vi "Ion Sniffer NXG.vi"() -> ()   [LabVIEW 2018]
uses:
  Type Defs/Main States.ctl
  Type Defs/Open IPF.ctl
  Type Defs/Log Command.ctl
  Type Defs/RT Command.ctl
  FGVs/Global Variables.vi
  <vilib>/Utility/config.llb/Read Key (Path).vi
  <vilib>/Utility/config.llb/Write Key (Path).vi
  <vilib>/Utility/config.llb/Read Key (String).vi
  <vilib>/Utility/config.llb/Write Key (String).vi
  <vilib>/Utility/config.llb/Read Key (Boolean).vi
  <vilib>/Utility/error.llb/Error Cluster From Error Code.vi
  <vilib>/ErrorRing/Error Ring.xnode
  <vilib>/Utility/config.llb/NI_LVConfig.lvlib
panel:
  out "ItemTag":string
  in  "Stop":bool
  out "Error Out":errorcluster
  in  "Display":bool
  in  "Acquisition":bool
  in  "Tuning":bool
  in  "Diagnostics":bool
  in  "Configuration":bool
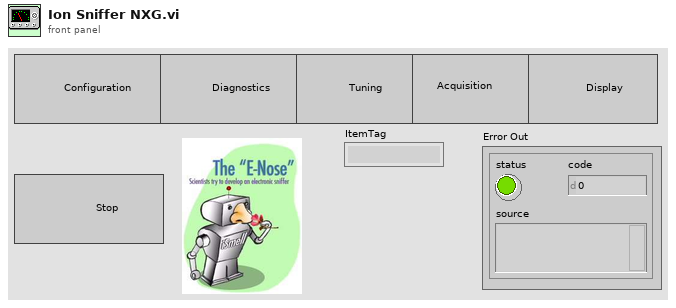
[diagram p1: front panel]
types:
  T1 = typedef "Main States.ctl" = enum16{"Initialize", "Init 2", "RT Stauts", "Exit"}
  T2 = typedef "Log Command.ctl" = enum16{"Close", "Write", "Open", "No Command"}
  T3 = typedef "Open IPF.ctl" = enum16{"Init", "Create IPF"}
  T4 = typedef "RT Command.ctl" = enum16{"xml Start Run", "xml Start Actual Run", "xml Stop Run", "xml Runtime Update", "xml Get Status", "xml Get Table", "xml Set Table", "xml Get Configuration", "xml System Status", "xml Set LC Input Logic", "xml Get Data", "xml Get Info", "Start", "StartActualRun", "Stop", "Runtime Update", "Get Data", "Get Info", "Get Status", "Get Param", "Get Config", "Get Table", "Read ADC", "Set Oscillator", "Update Config", "Update Table", "Set All Pol", "Set Pol and DC", "Set Max Mass", "Toggle RP", "Toggle EL", "Set PIC", "Initialize Turbo", "Send Turbo Comm", "Close Turbo", "P1", "P2", "P3", "Send Serial", "Set LC Out", "Get LC In", "Read VAC", "Test Table", "Toggle Power", "Get Startup", "Set Startup", "Get ADC Table", "Set ADC Table", "Get Brief Status", "Get Detail Status", "Auxiliary Update", "Set CC Logics", "Set CC Input Logics", "Ignore Error", "invalid"}
  T5 = typedef "NI_LVConfig.lvlib/Config Data RefNum.ctl" = refnum<k1>
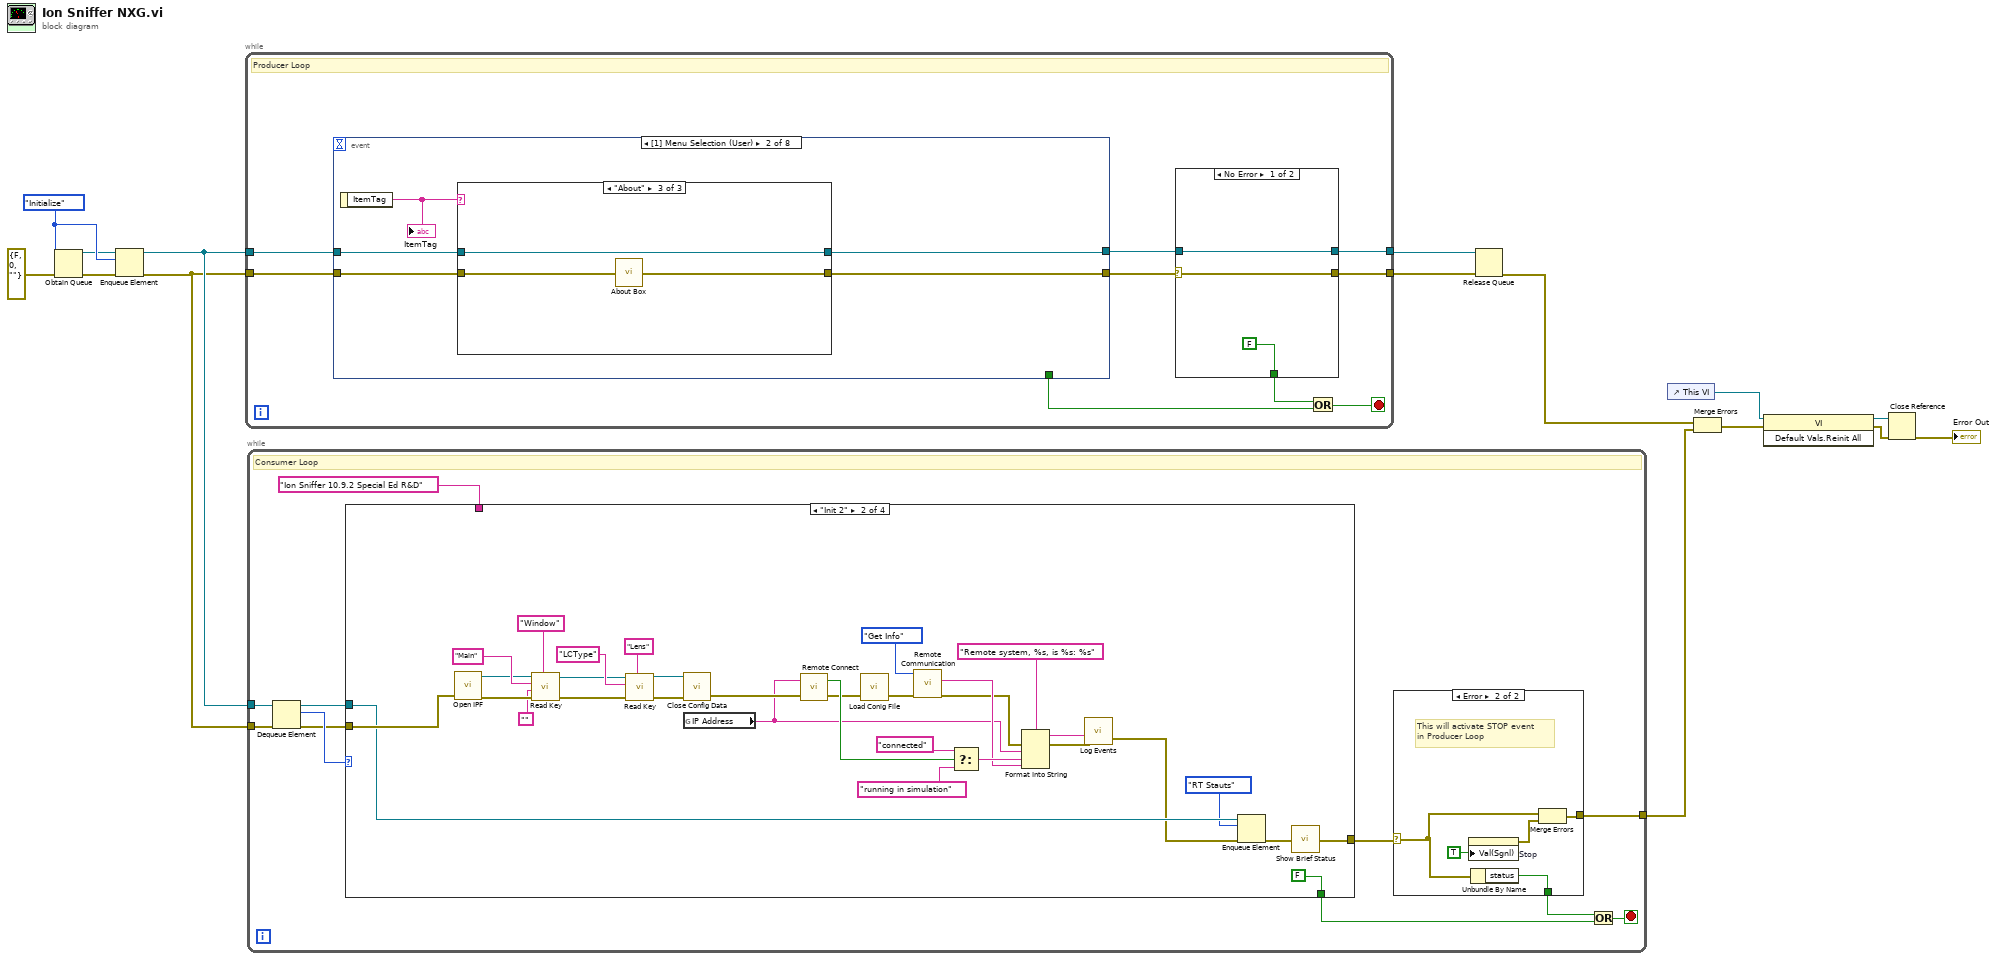
[diagram p0: block diagram]
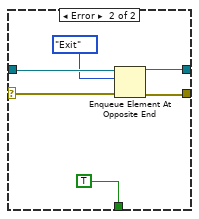
[diagram p2: hidden frame]
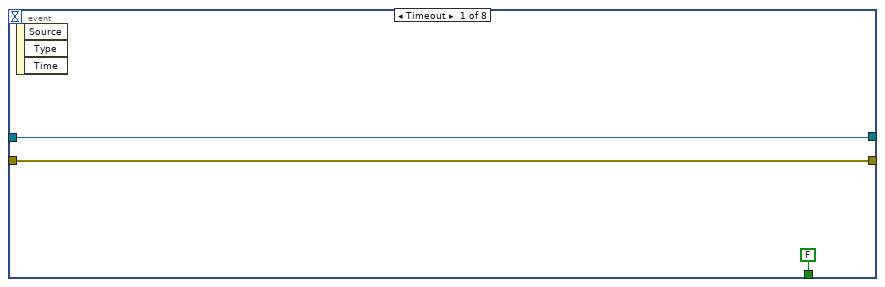
[diagram p3: hidden frame]
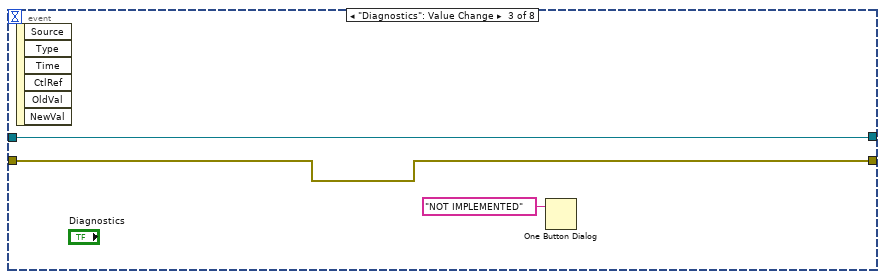
[diagram p6: hidden frame]
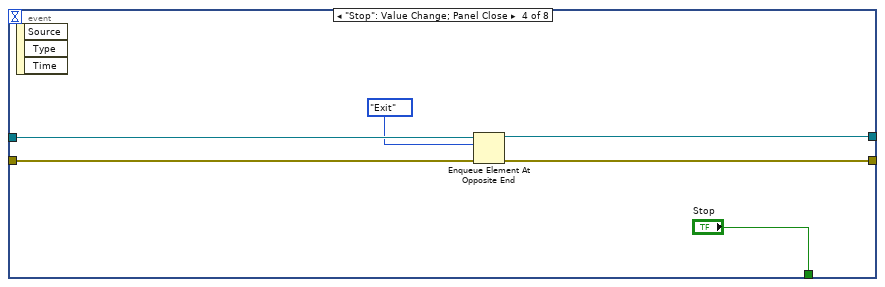
[diagram p7: hidden frame]
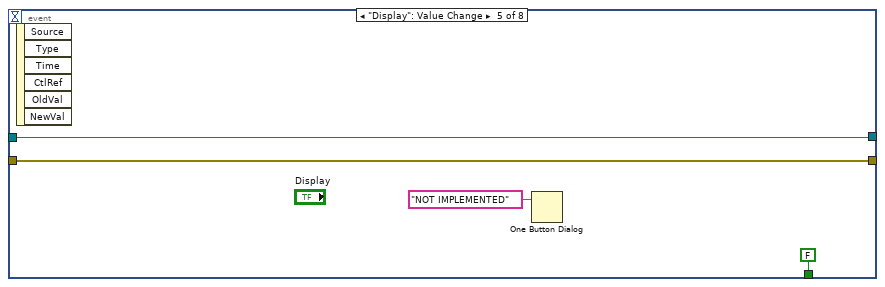
[diagram p8: hidden frame]
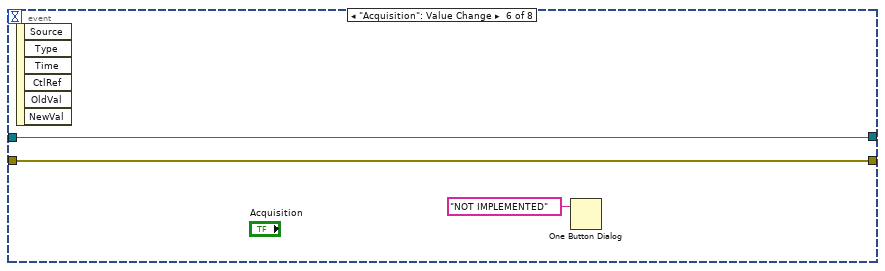
[diagram p9: hidden frame]
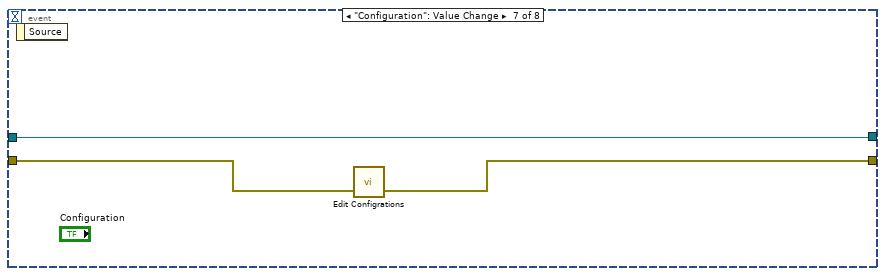
[diagram p10: hidden frame]
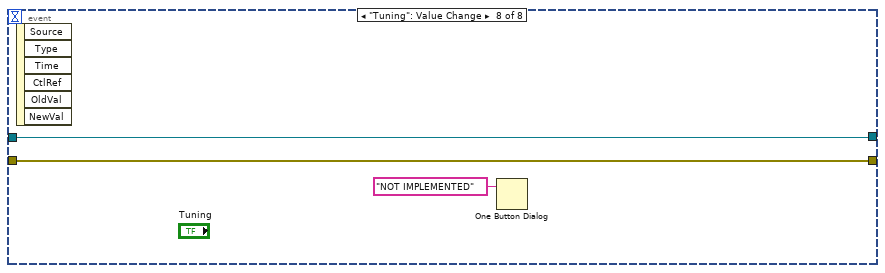
[diagram p11: hidden frame]
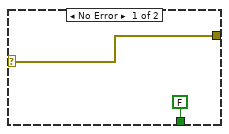
[diagram p12: hidden frame]
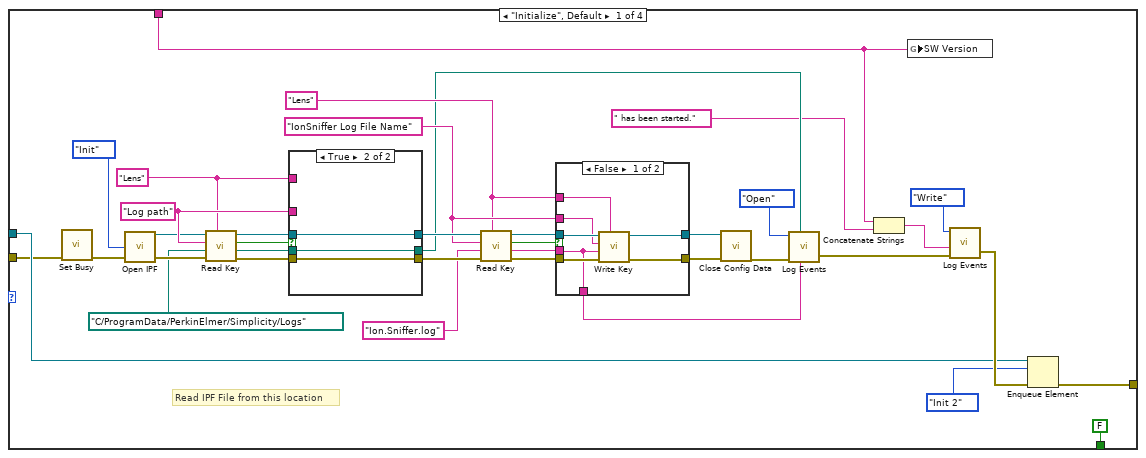
[diagram p13: hidden frame]
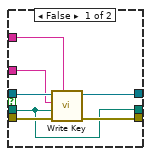
[diagram p15: hidden frame]
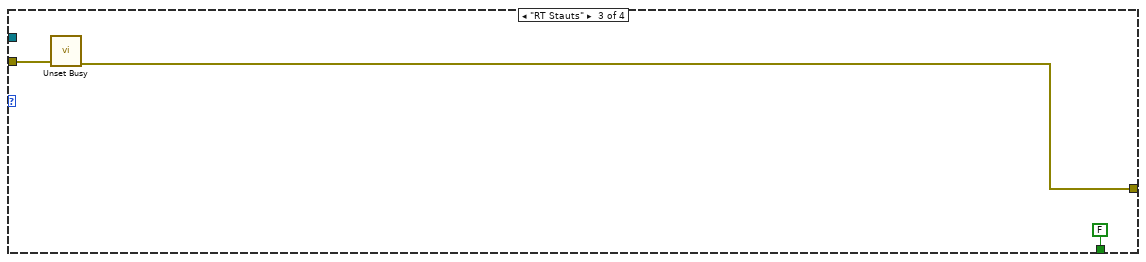
[diagram p16: hidden frame]
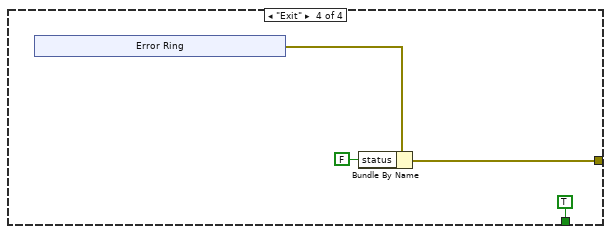
[diagram p17: hidden frame]
diagram:
  w15 = Main_States."Initialize"
  n1 = Obtain Queue(element data type=w15, error in (no error)=errorcluster {"status"=FALSE, "code"=0, "source"=""} ("error constant")) -> (queue out=w14:refnum<queue>, error out=w13:errorcluster)  [unwired: 3 in, 1 out]
  n2 = Enqueue Element(queue=w14, element=w15, error in (no error)=w13) -> (queue out=w11:refnum<queue>, error out=w10:errorcluster)  [unwired: 1 in, 1 out]
  n3 = while {
    tunnel: w11 -> [w23]
    tunnel: w10 -> [w24]
    tunnel: [w21] -> w9
    tunnel: [w19] -> w8
    stop <- w18 stop-if-true
    # "Producer Loop"
    n4 = event shown="[1] Menu Selection (User)" {
      selector: _ -> [_ _ _ _ _ _ _ _]
      dyn-events: _ -> [_ _ _ _ _ _ _ _]
      timeout: _ -> [_ _ _ _ _ _ _ _]
      tunnel: [FALSE ("Stop") _ _ "Stop" FALSE ("Stop") _ _ _] -> w16
      tunnel: w24 -> [w35 w40 w50 w56 w61 w64 w65 w70]
      tunnel: w23 -> [w36 w38 w51 w55 w60 w63 w67 w69]
      tunnel: [w35 w39 w50 w53 w61 w64 w66 w70] -> w22
      tunnel: [w36 w37 w51 w52 w60 w63 w67 w69] -> w20
      event Timeout {
        n5 = event-data() -> ()  [unwired: 1 in, 3 out]
      }
      event Menu Selection (User) {
        n6 = event-data() -> ("ItemTag"=w41:string)  [unwired: 1 in]
        "ItemTag" <- w41
        n7 = case shown="\"About\"" w41 {
          tunnel: w40 -> [w42 w44 w47]
          tunnel: [w42 w44 w46] -> w39
          tunnel: w38 -> [w43 w45 w48]
          tunnel: [w43 w45 w48] -> w37
          frame "False", Default {
          }
          frame "CH Test" {
          }
          frame "About" {
            n8 = call "About Box.vi"("error in (no error)"=w47) -> ("error out"=w46:errorcluster)
          }
        }
      }
      event "Diagnostics": Value Change {
        n9 = event-data() -> ()  [unwired: 1 in, 6 out]
        n10 = One Button Dialog(message="NOT IMPLEMENTED") -> ()  [unwired: 1 in, 1 out]
      }
      event "Stop": Value Change; Panel Close {
        n11 = event-data() -> ()  [unwired: 1 in, 3 out]
        n12 = Enqueue Element At Opposite End(queue=w55, element=Main_States."Exit", error in (no error)=w56) -> (queue out=w52:refnum<queue>, error out=w53:errorcluster)  [unwired: 1 in, 1 out]
      }
      event "Display": Value Change {
        n13 = event-data() -> ()  [unwired: 1 in, 6 out]
        n14 = One Button Dialog(message="NOT IMPLEMENTED") -> ()  [unwired: 1 in, 1 out]
      }
      event "Acquisition": Value Change {
        n15 = event-data() -> ()  [unwired: 1 in, 6 out]
        n16 = One Button Dialog(message="NOT IMPLEMENTED") -> ()  [unwired: 1 in, 1 out]
      }
      event "Configuration": Value Change {
        n17 = event-data() -> ()  [unwired: 1 in, 1 out]
        n18 = call "Edit Configrations.vi"("Error In"=w65) -> ("Error Out"=w66:errorcluster)  [unwired: 2 in]
      }
      event "Tuning": Value Change {
        n19 = event-data() -> ()  [unwired: 1 in, 6 out]
        n20 = One Button Dialog(message="NOT IMPLEMENTED") -> ()  [unwired: 1 in, 1 out]
      }
    }
    n21 = case shown="No Error" w22 {
      selector: w22 -> [w27 w30]
      tunnel: [w27 w32] -> w21
      tunnel: w20 -> [w26 w33]
      tunnel: [w26 w31] -> w19
      tunnel: [FALSE TRUE] -> w17
      frame No Error {
      }
      frame Error {
        n22 = Enqueue Element At Opposite End(queue=w33, element=Main_States."Exit", error in (no error)=w30) -> (queue out=w31:refnum<queue>, error out=w32:errorcluster)  [unwired: 1 in, 1 out]
      }
    }
    n23 = Or(x=w17, y=w16) -> (x .or. y?=w18:bool)
  }
  n24 = while {
    tunnel: w11 -> [w81]
    tunnel: w10 -> [w80]
    tunnel: [w74] -> w7
    stop <- w73 stop-if-true
    # "Consumer Loop"
    n25 = Dequeue Element(queue=w81, error in (no error)=w80) -> (queue out=w77:refnum<queue>, element=w79:T1, error out=w78:errorcluster)  [unwired: 1 in, 1 out]
    n26 = case shown="\"Init 2\"" w79 {
      tunnel: w78 -> [w90 w177 w179 _]
      tunnel: w77 -> [w96 w174 _ _]
      tunnel: "Ion Sniffer 10.9.2 Special Ed R&D" ("string") -> [w91 _ _ _]
      tunnel: [w95 w176 w178 w182] -> w75
      tunnel: [FALSE ("Value (Signaling)") FALSE ("Value (Signaling)") FALSE ("Value (Signaling)") TRUE ("Value (Signaling)")] -> w71
      frame "Initialize", Default {
        w108 = "Lens" ("section")
        w109 = "IonSniffer Log File Name" ("key")
        w117 = "Lens" ("section")
        w118 = "Log path" ("key")
        # "Read IPF File from this location"
        n27 = call <vilib>:"Set Busy.vi"("error in (no error)"=w90) -> ("error out"=w89:errorcluster)  [unwired: 9 in, 1 out]
        n28 = call "Open IPF.vi"("Error In"=w89, 4:Open_IPF."Init") -> ("Error Out"=w124:errorcluster, "IPF refnum"=w92:T5)  [unwired: 1 in, 1 out]
        n29 = call-poly <vilib>:"Read Key.vi"("section"=w117, "error in (no error)"=w124, "default value"=path "C:/ProgramData/PerkinElmer/Simplicity/Logs", "key"=w118, "refnum"=w92) -> ("error out"=w122:errorcluster, "value"=w119:path, "found?"=w121:bool, "refnum out"=w120:T5)  [unwired: 3 in]
        n30 = case shown="True" w121 {
          tunnel: w122 -> [w142 w145]
          tunnel: w119 -> [w136 w143]
          tunnel: w120 -> [w140 w144]
          tunnel: [w141 w145] -> w116
          tunnel: [w139 w144] -> w115
          tunnel: [w136 w143] -> w100
          tunnel: w117 -> [w138 _]
          tunnel: w118 -> [w137 _]
          frame False {
            n31 = call-poly <vilib>:"Write Key.vi"("section"=w138, "error in (no error)"=w142, "value"=w136, "key"=w137, "refnum"=w140) -> ("error out"=w141:errorcluster, "refnum out"=w139:T5)  [unwired: 4 in, 1 out]
          }
          frame True {
          }
        }
        n32 = call-poly <vilib>:"Read Key.vi"("section"=w108, "error in (no error)"=w116, "default value"="Ion.Sniffer.log", "key"=w109, "refnum"=w115) -> ("error out"=w113:errorcluster, "value"=w110:string, "found?"=w112:bool, "refnum out"=w111:T5)  [unwired: 3 in]
        n33 = case shown="False" w112 {
          tunnel: w113 -> [w132 w135]
          tunnel: w110 -> [w126 w133]
          tunnel: w111 -> [w130 w134]
          tunnel: [w131 w135] -> w107
          tunnel: [w129 w134] -> w106
          tunnel: w108 -> [w128 _]
          tunnel: w109 -> [w127 _]
          tunnel: [w126 w133] -> w104
          frame False {
            n34 = call-poly <vilib>:"Write Key.vi"("section"=w128, "error in (no error)"=w132, "value"=w126, "key"=w127, "refnum"=w130) -> ("error out"=w131:errorcluster, "refnum out"=w129:T5)  [unwired: 4 in, 1 out]
          }
          frame True {
          }
        }
        n35 = call <vilib>:"Close Config Data.vi"("error in (no error)"=w107, "refnum"=w106) -> ("error out"=w103:errorcluster)  [unwired: 1 in, 8 out]
        n36 = call "Log Events.vi"("File Name"=w104, "Log Path"=w100, "Error In"=w103, "Log Command"=Log_Command."Open") -> ("Error Out"=w102:errorcluster)  [unwired: 2 in, 1 out]
        n37 = Concatenate Strings(w91, " has been started." ("string")) -> (w98:string)
        n38 = global write "Global Variables.vi" "SW Version"(w91) -> ()
        n39 = call "Log Events.vi"("Error In"=w102, "Event"=w98, "Log Command"=Log_Command."Write") -> ("Error Out"=w97:errorcluster)  [unwired: 3 in, 1 out]
        n40 = Enqueue Element(queue=w96, element=Main_States."Init 2", error in (no error)=w97) -> (error out=w95:errorcluster)  [unwired: 1 in, 2 out]
      }
      frame "Init 2" {
        n41 = call "Open IPF.vi"("Error In"=w177) -> ("Error Out"=w172:errorcluster, "IPF refnum"=w153:T5)  [unwired: 2 in, 1 out]
        n42 = call-poly <vilib>:"Read Key.vi"("section"="Window", "error in (no error)"=w172, "default value"="", "key"="Main" ("section"), "refnum"=w153) -> ("error out"=w151:errorcluster, "refnum out"=w150:T5)  [unwired: 1 in, 4 out]
        n43 = call-poly <vilib>:"Read Key.vi"("section"="Lens", "error in (no error)"=w151, "key"="LCType" ("section"), "refnum"=w150) -> ("error out"=w167:errorcluster, "refnum out"=w166:T5)  [unwired: 1 in, 5 out]
        n44 = call <vilib>:"Close Config Data.vi"("error in (no error)"=w167, "refnum"=w166) -> ("error out"=w165:errorcluster)  [unwired: 1 in, 8 out]
        n45 = global read "Global Variables.vi" "IP Address"() -> (w149:string)
        n46 = call "Remote Connect.vi"("Error In"=w165, "IP Address"=w149) -> ("Error Out"=w147:errorcluster, "TCP"=w161:bool)
        n47 = call "Load Conig File.vi"("error in (no error)"=w147) -> ("error out"=w148:errorcluster)  [unwired: 1 in, 1 out]
        n48 = call "Remote Communication.vi"("Error In"=w148, "Command"=RT_Command."Get Info") -> ("Error Out"=w158:errorcluster, "Info"=w159:string)  [unwired: 4 in, 2 out]
        n49 = Select(t="connected", s=w161, f="running in simulation") -> (s? t:f=w164:string)
        n50 = Format Into String(format string="Remote system, %s, is %s: %s", error in=w158, w149, w164, w159) -> (resulting string=w157:string, error out=w156:errorcluster)  [unwired: 1 in]
        n51 = call "Log Events.vi"("Error In"=w156, "Event"=w157) -> ("Error Out"=w155:errorcluster)  [unwired: 4 in, 1 out]
        n52 = Enqueue Element(queue=w174, element=Main_States."RT Stauts", error in (no error)=w155) -> (error out=w175:errorcluster)  [unwired: 1 in, 2 out]
        n53 = call "Show Brief Status.vi"("Error In"=w175) -> ("Error Out"=w176:errorcluster)
      }
      frame "RT Stauts" {
        n54 = call <vilib>:"Unset Busy.vi"("error in (no error)"=w179) -> ("error out"=w178:errorcluster)  [unwired: 1 in, 9 out]
      }
      frame "Exit" {
        n55 = xnode "Error Ring"() -> ("error out"=w183:errorcluster)
        n56 = Bundle By Name(cluster=w183, "status"=FALSE) -> (w182:errorcluster)
      }
    }
    n57 = case shown="Error" w75 {
      selector: w75 -> [w83 w84]
      tunnel: [w83 w86] -> w74
      tunnel: [FALSE w88] -> w72
      frame No Error {
      }
      frame Error {
        # "This will activate STOP event \nin Producer Loop"
        n58 = property on="Stop" class="Bool (strict)"("Val(Sgnl)"=TRUE ("Value (Signaling)")) -> (error out=w85:errorcluster)  [unwired: 2 in, 1 out]
        n59 = Unbundle By Name(w84) -> ("status"=w88:bool)
        n60 = Merge Errors(w84, w85) -> (w86:errorcluster)
      }
    }
    n61 = Or(x=w72, y=w71) -> (x .or. y?=w73:bool)
  }
  n62 = Release Queue(queue=w8, error in (no error)=w9) -> (error out=w6:errorcluster)  [unwired: 1 in, 2 out]
  n63 = control-ref of="This VI"() -> (w5:refnum<vi>)
  n64 = Merge Errors(w6, w7) -> (w4:errorcluster)
  n65 = invoke class="VI" method="Default Vals.Reinit All"(reference=w5, error in=w4) -> (reference out=w2:refnum<vi>, error out=w3:errorcluster)  [unwired: 1 in, 1 out]
  n66 = Close Reference(reference=w2, error in (no error)=w3) -> (error out=→"Error Out":errorcluster)
